vi "PF_Slete.vi"(8 "error in (no error)":errorcluster caption="错误输入（无错误）", 11 "All_Result":bool[](array[boolean])) -> (0 "error out":errorcluster caption="错误输出", 3 "字符串":string)   [LabVIEW 2018]
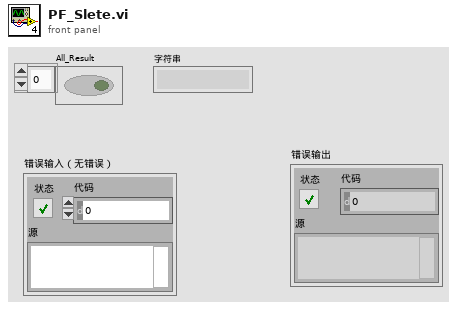
[diagram p1: front panel]
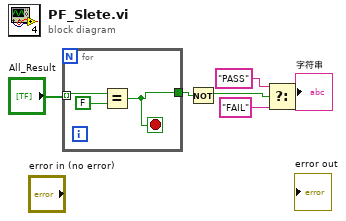
[diagram p0: block diagram]
diagram:
  n1 = for {
    tunnel: "All_Result" -> [w9] mode=indexing
    tunnel: [w7] -> w1
    stop <- w7 stop-if-true
    n2 = Equal?(x=w9, y=FALSE) -> (x = y?=w7:bool)
  }
  n3 = Not(x=w1) -> (.not. x?=w4:bool)
  n4 = Select(t="PASS" ("字符串"), s=w4, f="FAIL" ("字符串")) -> (s? t:f=→"字符串":string)
